vi "pruebas_digw.vi"() -> ()   [LabVIEW 2025]
panel:
  in  "stop":bool
  out "read buffer":string
  in  "Pin":i8=4 min=4 max=39 step=1
  in  "Boolean":bool
  in  "VISA resource name":refnum<visa-resource-name>
  out "error out":errorcluster
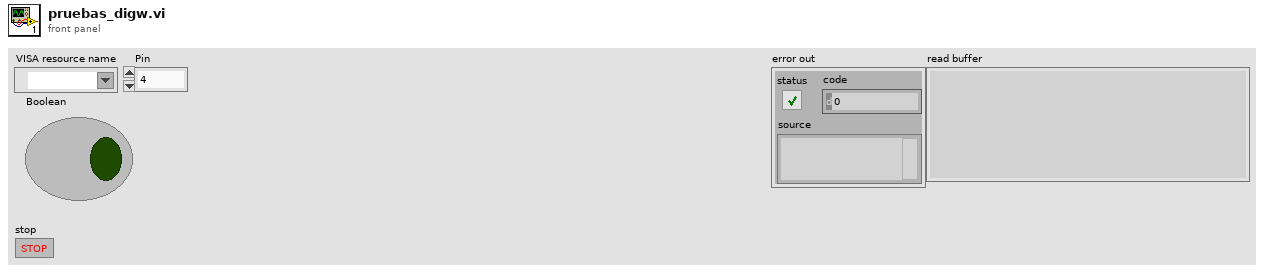
[diagram p1: front panel]
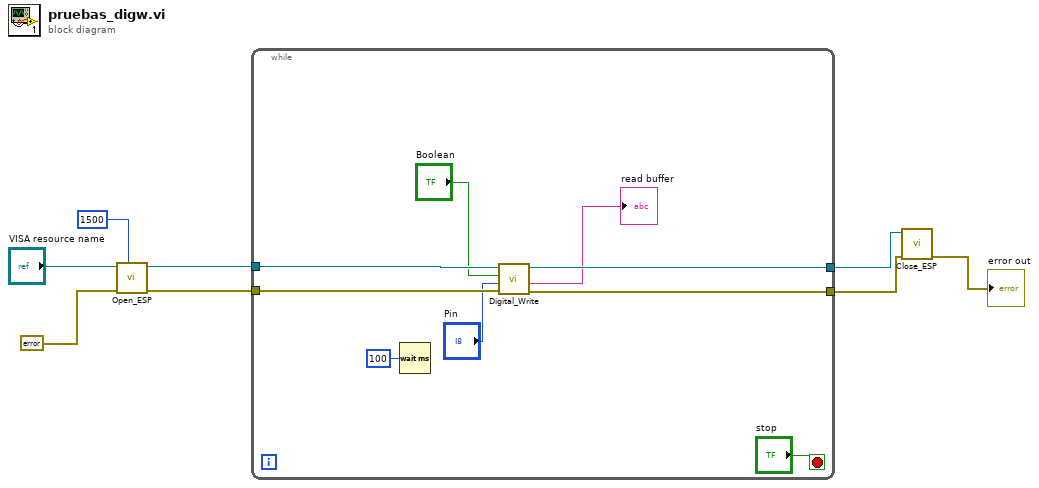
[diagram p0: block diagram]
diagram:
  n1 = call "Open_ESP.vi"("timeout (10sec)"=u32 1500, "error in (no error)"=errorcluster {"status"=FALSE, "code"=0, "source"=""}, "VISA resource name"="VISA resource name") -> ("error out"=w6:errorcluster, "VISA resource name out"=w8:refnum<visa-resource-name>)  [unwired: 7 in]
  n2 = while {
    tunnel: w8 -> [w16]
    tunnel: [w15] -> w7
    tunnel: w6 -> [w14]
    tunnel: [w13] -> w5
    stop <- "stop" stop-if-true
    n3 = Wait (ms)(milliseconds to wait=u32 100) -> ()  [unwired: 1 out]
    n4 = call "Digital_Write.vi"("error in (no error)"=w14, "Pin"="Pin", "Boolean"="Boolean", "VISA resource name"=w16) -> ("error out"=w13:errorcluster, "read buffer"=→"read buffer":string, "VISA resource name out"=w15:refnum<visa-resource-name>)  [unwired: 5 in]
  }
  n5 = call "Close_ESP.vi"("error in (no error)"=w5, "VISA resource name"=w7) -> ("error out"=→"error out":errorcluster)  [unwired: 9 in]
